vi "sendSetpointRequest.vi"(8 "error in (no error)":errorcluster, 10 "temperatureSetpoint":dbl[unit]=273.15, 11 "Model in":refnum<class "Model.lvclass">) -> (0 "error out":errorcluster, 3 "Model out":refnum<class "Model.lvclass">)   [LabVIEW 2013, in "Model.lvclass"]
uses:
  Model.lvclass
  Model.lvclass/Model.ctl
  UserEvents/UserEvents.lvclass/UserEvents.ctl
  ApplicationElements/Log/TestDataLog/TestDataLog.lvclass/TestDataLog.ctl
  UserEvents/UserEvents.lvclass
  ApplicationElements/Log/TestDataLog/TestDataLog.lvclass
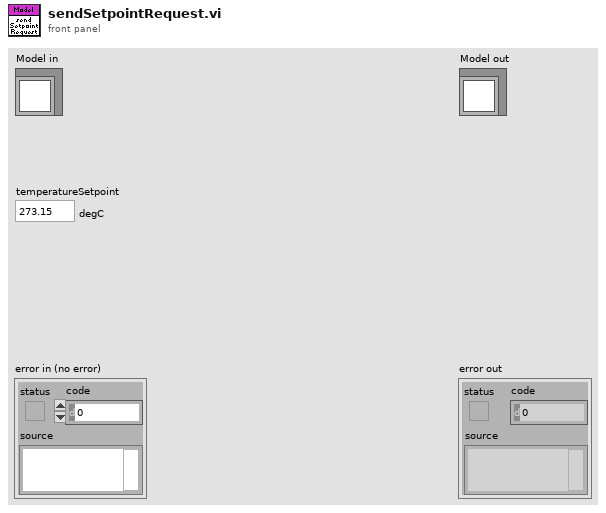
[diagram p1: front panel]
types:
  T1 = typedef "AITDTTypedefs.lvlib/PubDataEvents.ctl" = cluster{"State":refnum<user-event>, "ErrorCode":refnum<user-event>, "OutputData":refnum<user-event>, "InputData":refnum<user-event>, "TestStatus":refnum<user-event>, "LogPath":refnum<user-event>, "TemperatureSetpointRequest":refnum<user-event>}
  T2 = typedef "AITDTTypedefs.lvlib/TestStatus.ctl" = cluster{"activeCycle":u32, "activeProfileStep":u32, "demandedCycles":u32, "demandedProfileSteps":u32, "temperatureSetpoint":dbl[unit], "pgaGainCoefficient":u16}
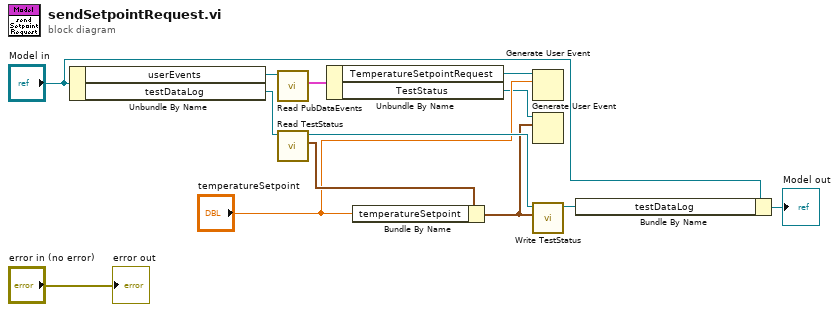
[diagram p0: block diagram]
diagram:
  n1 = Unbundle By Name("Model in") -> ("userEvents"=w12:refnum<class "UserEvents.lvclass">, "testDataLog"=w8:refnum<class "TestDataLog.lvclass">)
  n2 = call "Read PubDataEvents.vi"("UserEvents in"=w12) -> ("PubDataEvents"=w11:T1)  [unwired: 9 in, 1 out]
  n3 = call "Read TestStatus.vi"("Logger in"=w8) -> ("TestStatus"=w7:T2, "Logger out"=w6:refnum<class "TestDataLog.lvclass">)  [unwired: 9 in]
  n4 = Unbundle By Name(w11) -> ("TemperatureSetpointRequest"=w10:refnum<user-event>, "TestStatus"=w3:refnum<user-event>)
  n5 = Bundle By Name(cluster=w7, "temperatureSetpoint"="temperatureSetpoint") -> (w2:T2)
  n6 = Generate User Event(user event=w10, event data cluster="temperatureSetpoint") -> ()  [unwired: 2 in, 2 out]
  n7 = Generate User Event(user event=w3, event data cluster=w2) -> ()  [unwired: 2 in, 2 out]
  n8 = call "Write TestStatus.vi"("TestStatus"=w2, "Logger in"=w6) -> ("Logger out"=w4:refnum<class "TestDataLog.lvclass">)  [unwired: 9 in]
  n9 = Bundle By Name(cluster="Model in", "testDataLog"=w4) -> (→"Model out":refnum<class "Model.lvclass">)
  "error out" <- "error in (no error)"
